vi "Initialize milliGAT.vi"(10 "Enum in":refnum<vi>, 11 "VICI Settings in":T1) -> (0 "error out":errorcluster, 1 "error?":bool, 3 "VICI Settings out":T1)   [LabVIEW 2018, in "VICI M6 M50 Party Mode.lvlib"]
uses:
  VICI M6 M50 Party Mode.lvlib
  \\smbgbl.drmvfs102.pfizer.com\FAST_Team/Software/LabVIEW/Third Party Drivers/Third Party Drivers/VICI/Global FIA milliGAT.lvlib
  Settings Cluster.ctl
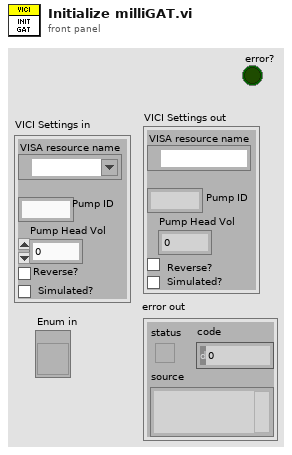
[diagram p1: front panel]
types:
  T1 = typedef "VICI M6 M50 Party Mode.lvlib/Settings Cluster.ctl" = cluster{"VISA resource name":refnum<visa-resource-name>, "Pump ID":string, "Pump Head Vol":dbl, "Reverse?":bool, "Simulated?":bool}
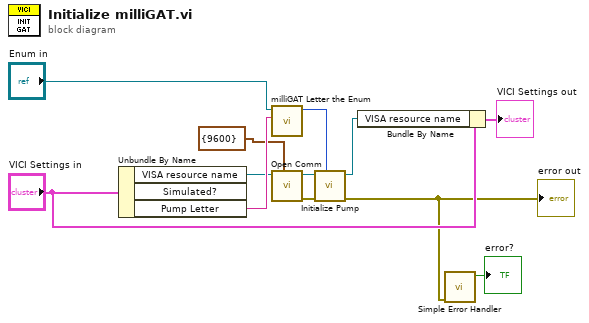
[diagram p0: block diagram]
diagram:
  n1 = Unbundle By Name("VICI Settings in") -> ("VISA resource name"=w5:refnum<visa-resource-name>, "Pump Letter"=w9:string)  [unwired: 1 out]
  n2 = call "milliGAT Letter the Enum.vi"("Pump Letter"=w9, "Enum in"="Enum in") -> ("Numeric"=w10:i32)  [unwired: 9 in]
  n3 = call "Open Comm.vi"("Serial Configuration"=cluster{"Baud Rate":u32} {"Baud Rate"=9600}, "VISA resource in"=w5) -> ("error out"=w8:errorcluster, "VISA resource out"=w7:refnum<visa-resource-name>)  [unwired: 8 in]
  n4 = call "Initialize Pump.vi"("Pump ID (0:A)"=w10, "error in (no error)"=w8, "VISA resource in"=w7) -> ("error out"=w2:errorcluster, "VISA resource out"=w12:refnum<visa-resource-name>)  [unwired: 7 in]
  "error out" <- w2
  n5 = Bundle By Name(cluster="VICI Settings in", "VISA resource name"=w12) -> (→"VICI Settings out":T1)
  n6 = call <vilib>:"Simple Error Handler.vi"("error in (no error)"=w2) -> ("error?"=→"error?":bool)  [unwired: 4 in, 4 out]
